vi "Acquisition Settings.vi"() -> ()   [LabVIEW 2009]
panel:
  in  "Signal Routing Configuration":T1(array[cluster]) {"Signal Routing"."signal source" items=["no change", "none", "AI start trigger", "AI stop trigger", "AI convert", "GPCTR 1 source", "GPCTR 1 gate", "AO update", "AO start trigger", "AI scan start", "GPCTR  0 source", "GPCTR  0 gate", "GPCTR  0 output", "RTSI 0", "RTSI 1", "RTSI 2", "RTSI 3", "RTSI 4", "RTSI 5", "RTSI 6", "RTSI clock", "board clock", "PLL input pin", "marker out", "SYNC out", "analog trigger circuit output", "end of acquisition", "frequency output", "high", "low", "SCANCLK", "inverted voltmeter complete", "voltmeter complete", "GPCTR n source", "GPCTR n gate", "GPCTR n output", "PFI n", "AI scan in progress", "(Reserved_1)", "(Reserved_2)", "stable 10MHz", "PXI Star"]; "Signal Routing"."signal name" items=["no change", "PFI 0", "PFI 1", "PFI 2", "PFI 3", "PFI 4", "PFI 5", "PFI 6", "PFI 7", "PFI 8", "PFI 9", "GPCTR 0 output", "RTSI 0", "RTSI 1", "RTSI 2", "RTSI 3", "RTSI 4", "RTSI 5", "RTSI 6", "RTSI clock", "board clock", "PLL reference clock", "SCANCLK", "I/O connector", "PFI n", "start trigger", "configurable filter", "PXI backplane clock", "PXI Star n"]}
  in  "Timer Settings":T2={"Device Number"=2, "Counter Number"=2, "Line Type for Source"=9, "Line Number for Source"=0, "Signal Routing Configuration"=0} {"Line Type for Source" items=["yes", "no", "positive", "negative", "high", "low", "low to high", "high to low", "default", "max timebase", "other counter gate", "other counter TC", "other counter output", "other counter source", "source", "gate", "aux line", "in start trigger", "in stop trigger", "automatic", "enabled", "count up", "count down", "hardware", "single", "double", "pulse", "toggle", "quadrature encoder X1", "quadrature encoder X2", "quadrature encoder X4", "two pulse counting", "A high B high", "A high B low", "A low B high", "A low B low", "PFI n", "RTSI n", "timebase n"]}
  in  "Pulse Generation Settings":T3(array[cluster])=[{"Name"="", "Device Number"=2, "Counter Number"=4, "Pulse Spec 1 (Clocks)"=40, "Pulse Spec 2 (Clocks)"=40, "Signal Routing Configuration"=0, "Inverted"=FALSE}]
  in  "AO Definitions":T4(array[cluster]) {"clock source (internal:1)" items=["no change", "internal", "counter 1", "counter 2", "counter 3", "counter 5", "I/O connector", "RTSI connection", "PFI pin, low to high", "PFI pin, high to low", "RTSI pin, low to high", "RTSI pin, high to low", "GPCTR 1 output, low to high", "GPCTR 1 output, high to low", "ATCOUT, low to high", "ACTOUT, high to low", "internal clock 2"]; "Signal Description"."period" format="%.2f"; "Signal Description"."% duty cycle" format="%.2f"; "Signal Description"."resting voltage" format="%.2f"; "Signal Description"."phase (0 deg)" format="%.2f"; "Signal Description"."offset (0.0)" format="%.2f"; "Signal Description"."amplitude" format="%.2f"}
  in  "Trigger Settings":T5={"Device Number"=2, "Counter Number"=3, "Signal Routing Configuration"=0}
  in  "Buffer Mode":u32(ring)=25 items=["yes", "no", "positive", "negative", "high", "low", "low to high", "high to low", "default", "max timebase", "other counter gate", "other counter TC", "other counter output", "other counter source", "source", "gate", "aux line", "in start trigger", "in stop trigger", "automatic", "enabled", "count up", "count down", "hardware", "single", "double", "pulse", "toggle", "quadrature encoder X1", "quadrature encoder X2", "quadrature encoder X4", "two pulse counting", "A high B high", "A high B low", "A low B high", "A low B low", "PFI n", "RTSI n", "timebase n"]
  in  "Arrival Time Settings":T6(array[cluster])=[{"Name"="Ch 1", "Device Number"=2, "Counter Number"=0, "Line Type for Gate"=36, "Line Number for Gate"=30, "Line Type for Source"=9, "Line Number for Source"=0, "Transfer Method"=47, "Signal Routing Configuration"=0}, {"Name"="Ch 2", "Device Number"=2, "Counter Number"=1, "Line Type for Gate"=36, "Line Number for Gate"=34, "Line Type for Source"=9, "Line Number for Source"=0, "Transfer Method"=47, "Signal Routing Configuration"=0}, {"Name"="Ch 3", "Device Number"=1, "Counter Number"=0, "Line Type for Gate"=36, "Line Number for Gate"=30, "Line Type for Source"=37, "Line Number for Source"=7, "Transfer Method"=47, "Signal Routing Configuration"=0}, {"Name"="Ch 4", "Device Number"=1, "Counter Number"=1, "Line Type for Gate"=36, "Line Number for Gate"=34, "Line Type for Source"=37, "Line Number for Source"=7, "Transfer Method"=47, "Signal Routing Configuration"=0}] {"Transfer Method" items=["yes", "no", "positive", "negative", "high", "low", "low to high", "high to low", "default", "max timebase", "other counter gate", "other counter TC", "other counter output", "other counter source", "source", "gate", "aux line", "in start trigger", "in stop trigger", "automatic", "enabled", "count up", "count down", "hardware", "single", "continuous", "pulse", "toggle", "quadrature encoder X1", "quadrature encoder X2", "quadrature encoder X4", "two pulse counting", "A high B high", "A high B low", "A low B high", "A low B low", "PFI n", "RTSI n", "timebase n", "disabled", "PXI backplane clock", "counter n output", "(Reserved) pulse per second", "(Reserved) IRIG-B", "(Reserved) seconds", "(Reserved) nano seconds", "interrupts", "dma", "RTSI clock"]; "Line Type for Source" items=["yes", "no", "positive", "negative", "high", "low", "low to high", "high to low", "default", "max timebase", "other counter gate", "other counter TC", "other counter output", "other counter source", "source", "gate", "aux line", "in start trigger", "in stop trigger", "automatic", "enabled", "count up", "count down", "hardware", "single", "double", "pulse", "toggle", "quadrature encoder X1", "quadrature encoder X2", "quadrature encoder X4", "two pulse counting", "A high B high", "A high B low", "A low B high", "A low B low", "PFI n", "RTSI n", "timebase n"]; "Line Type for Gate" items=["yes", "no", "positive", "negative", "high", "low", "low to high", "high to low", "default", "max timebase", "other counter gate", "other counter TC", "other counter output", "other counter source", "source", "gate", "aux line", "in start trigger", "in stop trigger", "automatic", "enabled", "count up", "count down", "hardware", "single", "double", "pulse", "toggle", "quadrature encoder X1", "quadrature encoder X2", "quadrature encoder X4", "two pulse counting", "A high B high", "A high B low", "A low B high", "A low B low", "PFI n", "RTSI n", "timebase n"]}
  in  "Buffer Size":i32=1000000
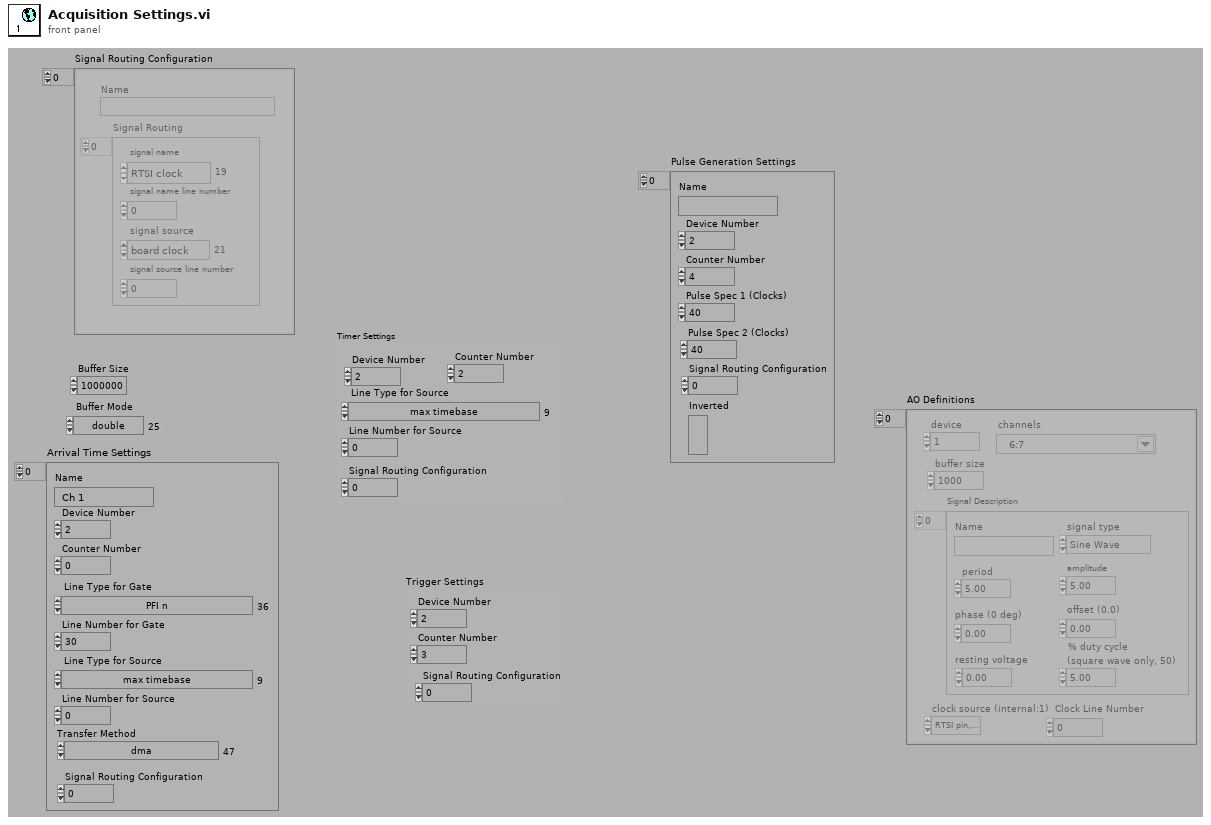
[diagram p1: front panel]
types:
  T1 = cluster{"Name":string, "Signal Routing":cluster{"signal name":u16, "signal source":u16, "signal source line number":u32, "signal name line number":u32}[]}[]
  T2 = cluster{"Device Number":i16, "Counter Number":i16, "Line Type for Source":u32, "Line Number for Source":u32, "Signal Routing Configuration":i16}
  T3 = cluster{"Name":string, "Device Number":i16, "Counter Number":i16, "Pulse Spec 1 (Clocks)":u32, "Pulse Spec 2 (Clocks)":u32, "Signal Routing Configuration":i16, "Inverted":bool}[]
  T4 = cluster{"device":i16, "channel":tag, "buffer size":i32, "Signal Description":cluster{"Name":string, "signal type":enum16{"Sine Wave", "Square Wave", "Sawtooth", "Triangle Wave"}, "period":dbl, "amplitude":dbl, "phase (0 deg)":dbl, "offset (0.0)":dbl, "resting voltage":dbl, "% duty cycle":dbl}[], "clock source (internal:1)":u16, "Clock Line Number":i16}[]
  T5 = cluster{"Device Number":i16, "Counter Number":i16, "Signal Routing Configuration":i16}
  T6 = cluster{"Name":string, "Device Number":i16, "Counter Number":i16, "Line Type for Gate":u32, "Line Number for Gate":u32, "Line Type for Source":u32, "Line Number for Source":u32, "Transfer Method":u32, "Signal Routing Configuration":i16}[]
diagram:
